vi "POS.vi"(0 "System no.":i32=1 min=1 max=4 step=1, 2 "Axes to set":string[](array[string]), 3 "Position values":dbl[](array[numeric]) format="%.6f", 4 "No.of digits":i16=4, 5 "error in":errorcluster) -> (19 "error out":errorcluster)   [LabVIEW 2020]
doc: "Assigns new position value to current position without moving the stage. Command can only be used when the reference mode is switched off (see RON.vi). No. of digits is the number of digits after the decimal point in the position value(s) that will be sent.\n\nWarning: If the current position is incorrectly set on an axis with reference mode OFF, the stage can be driven into the mechanical hard stop when moving to a position which is thought to be within the travel range of the stage, but actually is not.\n\nC-880K005: VI only supported when called through PI_Multix.vi\n\nE-755: Command not available for E-755.101\n\nE-861: With open-loop systems, this command is not useful because there is no position sensor."
panel:
  # "Assigns new position value to current position without moving the stage.\n\nWARNING: If the current position is incorrectly set on an axis with reference\nmode OFF, the stage can be driven into the mechanical hard stop when\nmoving to a position which is thought to be within the travel range of the\nstage, but actually is not!"
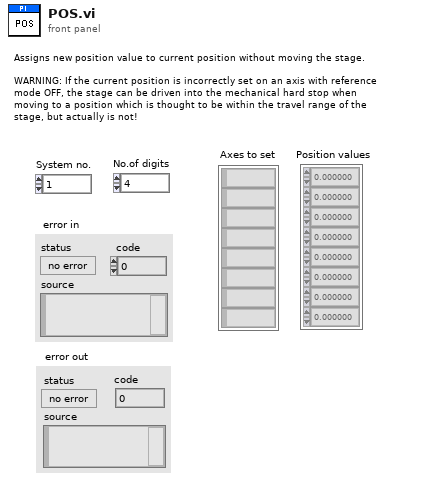
[diagram p1: front panel]
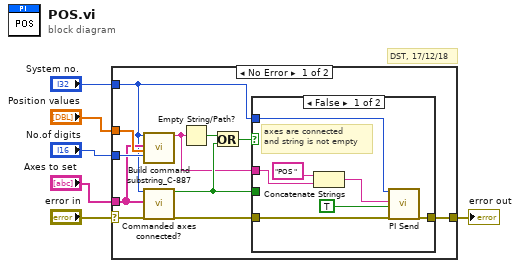
[diagram p0: block diagram]
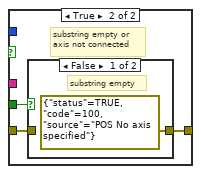
[diagram p2: hidden frame]
diagram:
  # "DST, 17/12/18"
  n1 = case shown="No Error" "error in" {
    selector: "error in" -> [w7 w30]
    tunnel: [w17 w30] -> w6
    tunnel: "Position values" -> [w16 _]
    tunnel: "No.of digits" -> [w15 _]
    tunnel: "System no." -> [w11 _]
    tunnel: "Axes to set" -> [w13 _]
    frame No Error {
      n2 = call "Build command substring_C-887.vi"("System no."=w11, "Affected axes"=w13, "Parameters"=w16, "No. of digits"=w15) -> ("Command substring"=w8:string)  [unwired: 3 in, 12 out]
      n3 = call "Commanded axes connected?.vi"("System no."=w11, "Commanded axes"=w13, "error in"=w7) -> ("Controller error"=w10:bool, "error out"=w14:errorcluster)  [unwired: 1 in, 14 out]
      n4 = Empty String/Path?(string/path=w8) -> (empty?=w9:bool)
      n5 = Or(x=w9, y=w10) -> (x .or. y?=w12:bool)
      n6 = case shown="False" w12 {
        tunnel: w8 -> [w23 _]
        tunnel: [w19 w27] -> w17
        tunnel: w14 -> [w20 w25]
        tunnel: w10 -> [_ w26]
        tunnel: w11 -> [w18 _]
        frame False {
          # "axes are connected \nand string is not empty"
          n7 = Concatenate Strings("POS ", w23) -> (w21:string)
          n8 = call "PI Send.vi"("System no."=w18, "String to send"=w21, "Attach termination char.?"=TRUE ("Attach Linefeed?"), "error in"=w20) -> ("error out"=w19:errorcluster)  [unwired: 2 in, 13 out]
        }
        frame True {
          # "substring empty or \naxis not connected"
          n9 = case shown="False" w26 {
            tunnel: [errorcluster {"status"=TRUE, "code"=100, "source"="POS No axis specified"} ("error out") w29] -> w27
            tunnel: w25 -> [_ w29]
            frame False {
              # "substring empty"
            }
            frame True {
              # "commanded axis \nnot connected"
            }
          }
        }
      }
    }
    frame Error {
    }
  }
  "error out" <- w6
